vi "InitializeStageOutputChannels.vi"(1 "1st Axis":u16(ring) items=["x", "y"]) -> (0 "Append Channels":tag)   [LabVIEW 2009]
panel:
  in  "VI Refnum":refnum<vi>
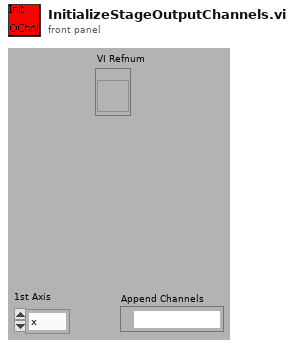
[diagram p1: front panel]
types:
  T1 = enum16{"Get Type", "Set Type", "GetStageInit", "GetWriteStageSetting", "GetInitializeStageOutput", "GetSetAxisPosition", "GetSetPos", "GetSetupStage", "HaltStageOutput", "InitializeStageOutputChannels"}
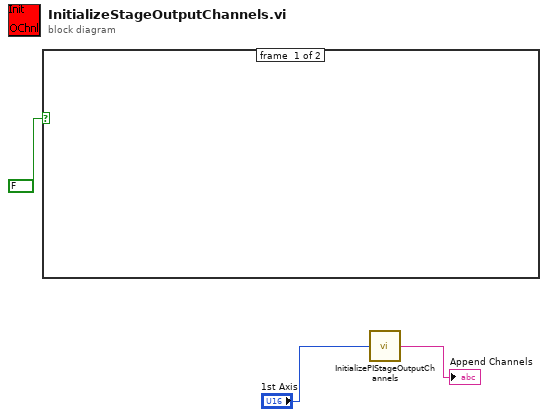
[diagram p0: block diagram]
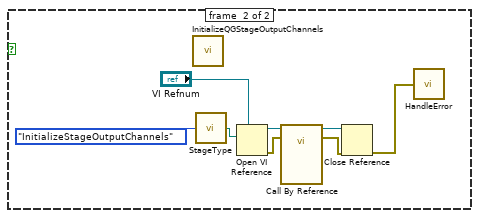
[diagram p2: hidden frame]
diagram:
  n1 = case shown="True" FALSE ("Case Constant\n(See Context Help)") {
    frame #0 {
    }
    frame #1 {
      n2 = call "InitializeQGStageOutputChannels.vi"() -> ()  [unwired: 1 in, 1 out]
      n3 = call "StageType.vi"("Function"=T1."InitializeStageOutputChannels") -> ("VI Path"=w4:path)  [unwired: 2 in, 2 out]
      n4 = Open VI Reference(type specifier VI Refnum (for type only)="VI Refnum", vi path=w4) -> (vi reference=w10:refnum<vi>, error out=w7:errorcluster)  [unwired: 4 in]
      n5 = call-by-ref "?"(reference=w10, error in=w7) -> (reference out=w6:refnum<vi>, error out=w8:errorcluster)  [unwired: 1 in, 1 out]
      n6 = Close Reference(reference=w6, error in (no error)=w8) -> (error out=w11:errorcluster)
      n7 = call "HandleError.vi"("error in (no error)"=w11) -> ()
    }
  }
  n8 = call "InitializePIStageOutputChannels.vi"("1st Axis"="1st Axis") -> ("Append Channels"=→"Append Channels":tag)
